vi "첫TDMS코딩_읽기.vi"() -> ()   [LabVIEW 2020]
uses:
  <vilib>/Utility/sysdir.llb/System Directory Type.ctl
panel:
  out "파형 신호":dbl[][](graph)
  out "전기 신호":dbl[][](graph)
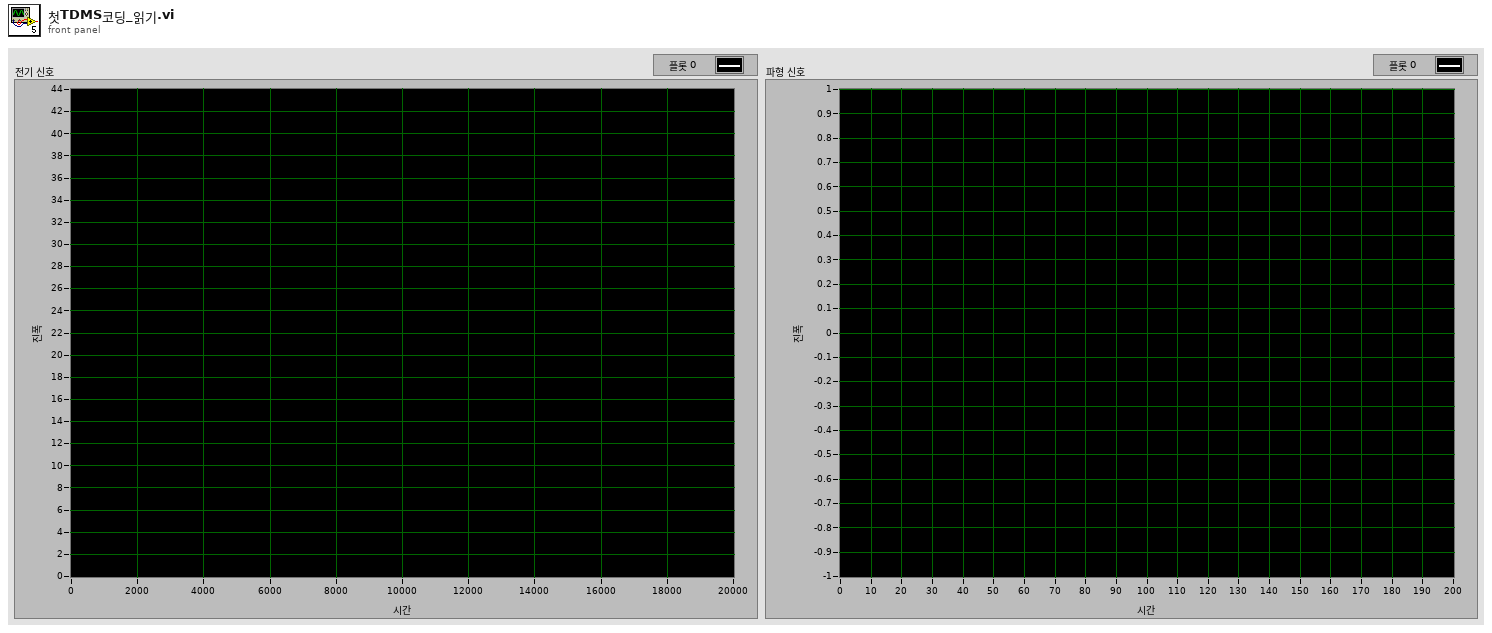
[diagram p1: front panel]
types:
  T1 = enum16{"open", "open or create", "create or replace", "create", "open (read-only)"}
  T2 = typedef "System Directory Type.ctl" = i32
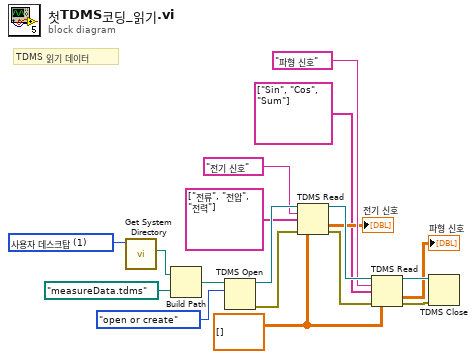
[diagram p0: block diagram]
diagram:
  w4 = dbl[][] []
  w18 = T2 1 items=["사용자 홈"=0, "사용자 데스크탑"=1, "사용자 문서"=2, "사용자 어플리케이션 데이터"=3, "사용자 환경"=4, "사용자 임시"=5, "퍼블릭 문서"=6, "퍼블릭 어플리케이션 데이터"=7, "퍼블릭 환경"=8, "퍼블릭 캐시"=13, "시스템 코어 라이브러리"=9, "시스템 설치된 라이브러리"=10, "어플리케이션 파일"=11, "부팅 볼륨 루트"=12] ("system directory type")
  # "TDMS 읽기 데이터"
  n1 = call <vilib>:"Get System Directory.vi"("system directory type"=w18) -> ("system directory"=w17:path)  [unwired: 10 in]
  n2 = Build Path(base path=w17, name or relative path=path "measureData.tdms" ("이름 또는 상대 경로")) -> (appended path=w15:path)
  n3 = TDMS Open(10:T1."open or create" ("동작(0:open)"), 11:w15) -> (0:w7:errorcluster, 3:w14:refnum<k34>)  [unwired: 5 in]
  n4 = TDMS Read(0:w14, 5:"전기 신호", 7:string[] ["전류", "전압", "전력"], 11:w7, 12:w4) -> (4:w13:refnum<k34>, 10:→"전기 신호":dbl[][], 15:w6:errorcluster)  [unwired: 3 in, 3 out]
  n5 = TDMS Read(0:w13, 5:"파형 신호", 7:string[] ["Sin", "Cos", "Sum"], 11:w6, 12:w4) -> (4:w12:refnum<k34>, 10:→"파형 신호":dbl[][], 15:w11:errorcluster)  [unwired: 3 in, 3 out]
  n6 = TDMS Close(8:w11, 11:w12) -> ()  [unwired: 2 out]
